vi "Teleop.vi"(10 "Match Info":T1={"Autonomous Elapsed Seconds"=0.0, "TeleOp Elapsed Seconds"=0.0, "Disabled Elapsed Seconds"=0.0, "Visited Autonomous"=FALSE, "Visited TeleOp"=FALSE, "Visited Disabled"=FALSE, "Autonomous Settings"={"Autonomous Style"=enum."Independent", "VI Refnum"=refnum}}, 11 "Call Context":T2) -> ()   [LabVIEW 2013]
doc: "This VI is called for each TeleOp packet received from the DS where the robot is not disabled. It is often used to read from the joysticks and update I/O or to update setpoints for timed control loops. It should complete and return within 20 milliseconds or it may miss DS packets."
uses:
  <vilib>/Rock Robotics/WPI/DriverStation/WPI_DriverStationDerivedRobotMode.ctl
  <vilib>/Rock Robotics/WPI/DriverStation/WPI_DriverStationMatch Info.ctl
  Robot Global Data.vi
  <vilib>/Rock Robotics/WPI/Joystick/WPI_JoystickGetSetRefNum.vi
  <vilib>/Rock Robotics/WPI/RobotDrive/WPI_RobotDriveGetSetRefNum.vi
  <vilib>/Rock Robotics/WPI/RobotDrive/WPI_RobotDriveArcadeDrive_Standard(NoSaturation).vi
panel:
  out "Angular Rate":dbl
  out "Angle":dbl
  out "Robot Moving?":bool
  out "Motor Values":dbl[](array[numeric])
  out "Numeric 1":dbl(slide) scale=0.0..100.0
  out "Boolean 2":bool
  out "Boolean 1":bool
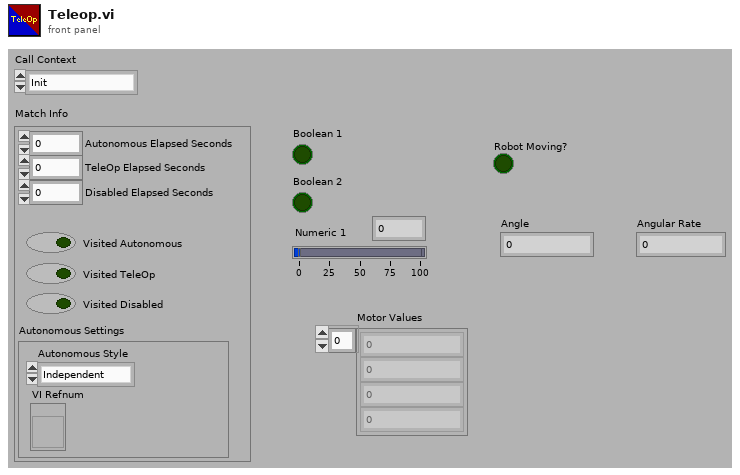
[diagram p1: front panel]
types:
  T1 = typedef "WPI_DriverStationMatch Info.ctl" = cluster{"Autonomous Elapsed Seconds":dbl, "TeleOp Elapsed Seconds":dbl, "Disabled Elapsed Seconds":dbl, "Visited Autonomous":bool, "Visited TeleOp":bool, "Visited Disabled":bool, "Autonomous Settings":cluster{"Autonomous Style":enum16{"Iterative", "Independent"}, "VI Refnum":refnum<vi>}}
  T2 = typedef "WPI_DriverStationDerivedRobotMode.ctl" = enum16{"Init", "Execute", "Stop"}
  T3 = typedef "WPI_JoystickDevRef.ctl" = cluster{"Device":T4}
  T4 = typedef "WPI_JoystickDeviceEnum.ctl" = enum16{"USB 1", "USB 2", "USB 3", "USB 4", "Kinect 1", "Kinect 2"}
  T5 = typedef "WPI_GyroDevRef.ctl" = cluster{"DevStatus":errorcluster, "Analog Module":T6, "Analog Channel":T7, "Offset":dbl, "Gain (VoltsPerDegree/Second)":dbl}
  T6 = typedef "FPGA_TypedefAnalogModule.ctl" = enum16{"Analog Module 1", "Analog Module 2"}
  T7 = typedef "FPGA_AIChannel.ctl" = enum8{"AI 1", "AI 2", "AI 3", "AI 4", "AI 5", "AI 6", "AI 7", "AI 8", "Invalid"}
  T8 = typedef "WPI_JoystickButtonState.ctl" = cluster{"Button 1":bool, "Button 2":bool, "Button 3":bool, "Button 4":bool, "Button 5":bool, "Button 6":bool, "Button 7":bool, "Button 8":bool, "Button 9":bool, "Button 10":bool, "Button 11":bool, "Button 12":bool}
  T9 = cluster{"axis 1 (x)":dbl, "axis 2 (y)":dbl, "axis 3 (throttle)":dbl, "axis 4":dbl, "axis 5":dbl, "axis 6":dbl}
  T10 = typedef "WPI_RobotDriveDevRef.ctl" = cluster{"DevStatus":errorcluster, "Motors[]":T11[], "Square Inputs":bool, "Max Output":dbl, "Isochronous":bool}
  T11 = typedef "WPI_MotorControlDeviceRef.ctl" = cluster{"DeviceStatus":errorcluster, "Type":enum16{"PWM", "CAN"}, "PWM":cluster{"Digital Module":T12, "PWM Channel":T13, "DeadBand":T14}, "CAN":cluster{"Device Number":u8, "Control Mode":T15, "Semaphore":T16, "Max Vout":dbl}, "Invert":bool, "TransformRef":T17, "InvTransformRef":T17}
  T12 = typedef "FPGA_TypedefDigitalModule.ctl" = enum16{"Digital Module 1", "Digital Module 2"}
  T13 = typedef "FPGA_DIOPWMChannel.ctl" = enum8{"PWM 1", "PWM 2", "PWM 3", "PWM 4", "PWM 5", "PWM 6", "PWM 7", "PWM 8", "PWM 9", "PWM 10", "Invalid"}
  T14 = typedef "WPI_PWMDeadband.ctl" = cluster{"Name":string, "maxPositivePwm":i32, "minPositivePwm":i32, "centerPwm":i32, "maxNegativePwm":i32, "minNegativePwm":i32, "angularRange":u16}
  T15 = typedef "WPI_CANJaguar_ControlMode.ctl" = enum8{"Percent VBus", "Current", "Speed", "Position", "Voltage"}
  T16 = typedef "Semaphore RefNum" = refnum<k1>
  T17 = typedef "WPI_PWMTransform_ConPane.ctl" = refnum<vi>
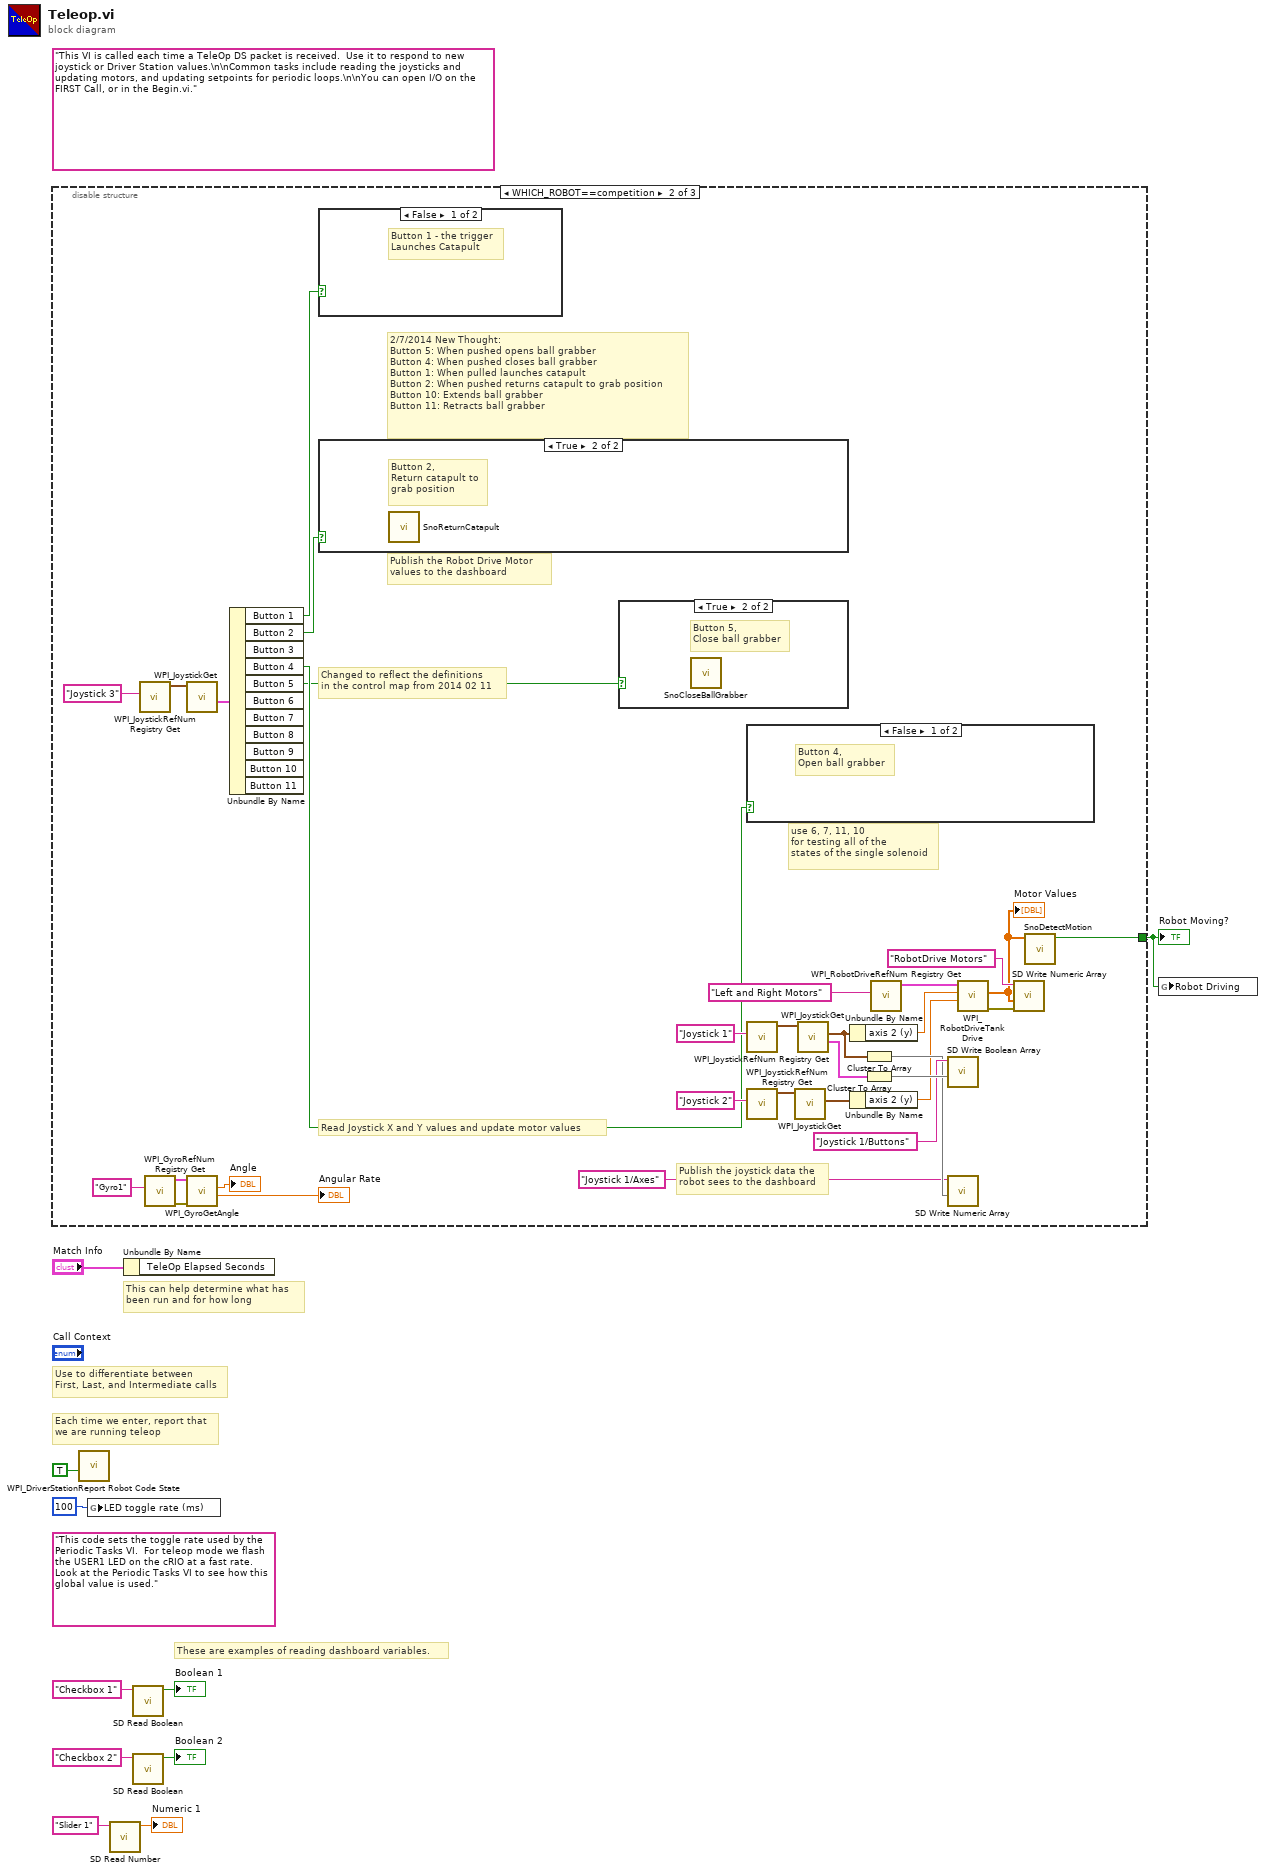
[diagram p0: block diagram]
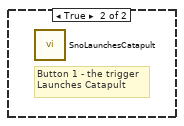
[diagram p4: hidden frame]
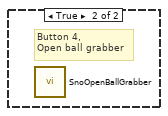
[diagram p5: hidden frame]
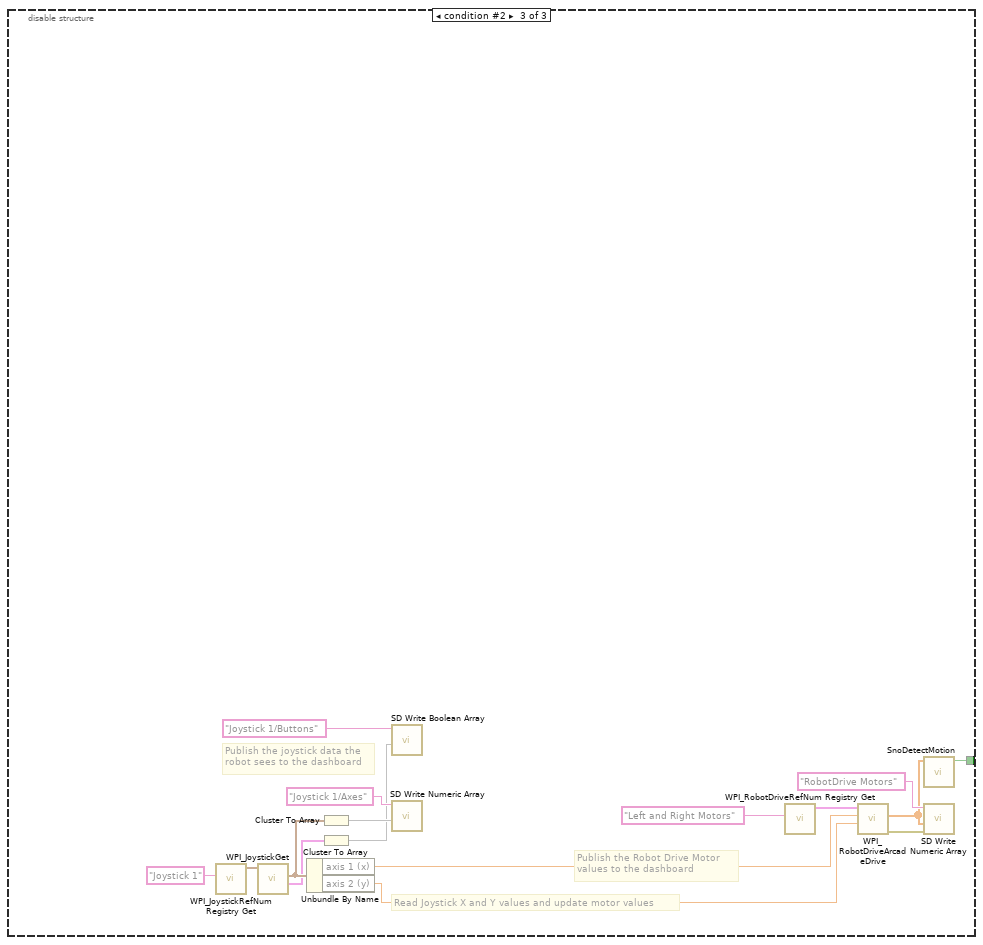
[diagram p7: hidden frame]
diagram:
  (unwired) "This code sets the toggle rate used by the Periodic Tasks VI.  For teleop mode we flash the USER1 LED on the cRIO at a fast rate.  Look at the Periodic Tasks VI to see how this global value is used."
  (unwired) "This VI is called each time a TeleOp DS packet is received.  Use it to respond to new joystick or Driver Station values.\n\nCommon tasks include reading the joysticks and updating motors, and updating setpoints for periodic loops.\n\nYou can open I/O on the FIRST Call, or in the Begin.vi."
  # "These are examples of reading dashboard variables."
  # "Each time we enter, report that\nwe are running teleop"
  # "Use to differentiate between\nFirst, Last, and Intermediate calls"
  # "This can help determine what has\nbeen run and for how long"
  n1 = disable-structure shown="WHICH_ROBOT==competition" {
    disable-tunnel: [_ w16 w42] -> w1
    frame condition #0 {
    }
    frame condition #1 (active) {
      # "use 6, 7, 11, 10\nfor testing all of the\nstates of the single solenoid"
      # "Changed to reflect the definitions\nin the control map from 2014 02 11"
      # "2/7/2014 New Thought:\nButton 5: When pushed opens ball grabber\nButton 4: When pushed closes ball grabber\nButton 1: When pulled launches catapult\nButton 2: When pushed returns catapult to grab position\nButton 10: Extends ball grabber\nButton 11: Retracts ball grabber"
      # "Publish the Robot Drive Motor\nvalues to the dashboard"
      # "Publish the joystick data the\nrobot sees to the dashboard"
      # "Read Joystick X and Y values and update motor values"
      n2 = call <vilib>:"WPI_JoystickRefNum Registry Get.vi"("refnum name"="Joystick 3") -> ("JoystickDevRef"=w25:T3)  [unwired: 1 in, 9 out]
      n3 = call <vilib>:"WPI_GyroRefNum Registry Get.vi"("refnum name"="Gyro1") -> ("error out"=w13:errorcluster, "GyroDevRef"=w14:T5)  [unwired: 9 in]
      n4 = call <vilib>:"WPI_JoystickGet.vi"("JoystickDevRef"=w25) -> ("Buttons"=w23:T8)  [unwired: 1 in, 5 out]
      n5 = call <vilib>:"WPI_GyroGetAngle.vi"("error in (no error)"=w13, "GyroDevRef"=w14) -> ("Angular Rate"=→"Angular Rate":dbl, "Angle"=→"Angle":dbl)  [unwired: 6 in, 2 out]
      n6 = Unbundle By Name(w23) -> ("Button 1"=w19:bool, "Button 2"=w18:bool, "Button 4"=w22:bool, "Button 5"=w21:bool)  [unwired: 7 out]
      n7 = case shown="False" w19 {
        frame False {
          # "Button 1 - the trigger\nLaunches Catapult"
        }
        frame True {
          # "Button 1 - the trigger\nLaunches Catapult"
          n8 = call "SnoLaunchesCatapult.vi"() -> ()  [unwired: 12 in]
        }
      }
      n9 = case shown="True" w18 {
        frame False {
          # "Button 2,\nReturn catapult to\ngrab position"
        }
        frame True {
          # "Button 2,\nReturn catapult to\ngrab position"
          n10 = call "SnoReturnCatapult.vi"() -> ()  [unwired: 12 in]
        }
      }
      n11 = case shown="True" w21 {
        frame False {
          # "Button 5,\nClose ball grabber"
        }
        frame True {
          # "Button 5,\nClose ball grabber"
          n12 = call "SnoCloseBallGrabber.vi"() -> ()  [unwired: 1 in, 2 out]
        }
      }
      n13 = case shown="False" w22 {
        frame False {
          # "Button 4,\nOpen ball grabber"
        }
        frame True {
          # "Button 4,\nOpen ball grabber"
          n14 = call "SnoOpenBallGrabber.vi"() -> ()  [unwired: 1 in, 1 out]
        }
      }
      n15 = call <vilib>:"WPI_JoystickRefNum Registry Get.vi"("refnum name"="Joystick 1") -> ("JoystickDevRef"=w39:T3)  [unwired: 1 in, 9 out]
      n16 = call <vilib>:"WPI_JoystickRefNum Registry Get.vi"("refnum name"="Joystick 2") -> ("JoystickDevRef"=w31:T3)  [unwired: 1 in, 9 out]
      n17 = call <vilib>:"WPI_JoystickGet.vi"("JoystickDevRef"=w31) -> ("Axes"=w30:T9)  [unwired: 1 in, 5 out]
      n18 = call <vilib>:"WPI_JoystickGet.vi"("JoystickDevRef"=w39) -> ("Buttons"=w20:T8, "Axes"=w36:T9)  [unwired: 1 in, 4 out]
      n19 = Unbundle By Name(w36) -> ("axis 2 (y)"=w28:dbl)
      n20 = Unbundle By Name(w30) -> ("axis 2 (y)"=w27:dbl)
      n21 = Cluster To Array(cluster=w36) -> (array=w35:dbl[])
      n22 = Cluster To Array(cluster=w20) -> (array=w38:bool[])
      n23 = call <vilib>:"WPI_RobotDriveRefNum Registry Get.vi"("refnum name"="Left and Right Motors") -> ("RobotDriveDevRef"=w29:T10)  [unwired: 1 in, 9 out]
      n24 = call <vilib>:"SD Write Boolean Array.vi"("Boolean Array"=w38, "Name"="Joystick 1/Buttons") -> ()  [unwired: 8 in, 2 out]
      n25 = call <vilib>:"SD Write Numeric Array.vi"("Numeric Array"=w35, "Name"="Joystick 1/Axes") -> ()  [unwired: 8 in, 2 out]
      n26 = call <vilib>:"WPI_RobotDriveTankDrive.vi"("Right axis value"=w27, "Left axis value"=w28, "RobotDriveDevRef"=w29) -> ("error out"=w26:errorcluster, "Motor Values"=w17:dbl[])  [unwired: 6 in, 1 out]
      "Motor Values" <- w17
      n27 = call <vilib>:"SD Write Numeric Array.vi"("error in"=w26, "Numeric Array"=w17, "Name"="RobotDrive Motors") -> ()  [unwired: 7 in, 2 out]
      n28 = call "SnoDetectMotion.vi"("Motor Values"=w17) -> ("Boolean"=w16:bool)  [unwired: 10 in]
    }
    frame condition #2 {
      # "Publish the Robot Drive Motor\nvalues to the dashboard"
      # "Publish the joystick data the\nrobot sees to the dashboard"
      # "Read Joystick X and Y values and update motor values"
      n29 = call <vilib>:"WPI_JoystickRefNum Registry Get.vi"("refnum name"="Joystick 1") -> ("JoystickDevRef"=w46:T3)  [unwired: 1 in, 9 out]
      n30 = call <vilib>:"WPI_JoystickGet.vi"("JoystickDevRef"=w46) -> ("Buttons"=w47:T8, "Axes"=w50:T9)  [unwired: 1 in, 4 out]
      n31 = Unbundle By Name(w50) -> ("axis 1 (x)"=w56:dbl, "axis 2 (y)"=w57:dbl)
      n32 = Cluster To Array(cluster=w50) -> (array=w51:dbl[])
      n33 = Cluster To Array(cluster=w47) -> (array=w48:bool[])
      n34 = call <vilib>:"SD Write Boolean Array.vi"("Boolean Array"=w48, "Name"="Joystick 1/Buttons") -> ()  [unwired: 8 in, 2 out]
      n35 = call <vilib>:"SD Write Numeric Array.vi"("Numeric Array"=w51, "Name"="Joystick 1/Axes") -> ()  [unwired: 8 in, 2 out]
      n36 = call <vilib>:"WPI_RobotDriveRefNum Registry Get.vi"("refnum name"="Left and Right Motors") -> ("RobotDriveDevRef"=w54:T10)  [unwired: 1 in, 9 out]
      n37 = call-poly <vilib>:"WPI_RobotDriveArcadeDrive.vi"("Y axis value"=w57, "X axis value"=w56, "RobotDriveDevRef"=w54) -> ("error out"=w55:errorcluster, "Motor Values"=w43:dbl[])  [unwired: 6 in, 1 out]
      n38 = call "SnoDetectMotion.vi"("Motor Values"=w43) -> ("Boolean"=w42:bool)  [unwired: 10 in]
      n39 = call <vilib>:"SD Write Numeric Array.vi"("error in"=w55, "Numeric Array"=w43, "Name"="RobotDrive Motors") -> ()  [unwired: 7 in, 2 out]
    }
  }
  "Robot Moving?" <- w1
  n40 = call <vilib>:"WPI_DriverStationReport Robot Code State.vi"("TeleOp"=TRUE ("Autonomous")) -> ()  [unwired: 10 in, 1 out]
  n41 = global write "Robot Global Data.vi" "LED toggle rate (ms)"(u32 100 ("LED ms toggle rate")) -> ()
  n42 = call <vilib>:"SD Read Number.vi"("Name"="Slider 1" ("refnum name")) -> ("Numeric"=→"Numeric 1":dbl)  [unwired: 8 in, 2 out]
  n43 = Unbundle By Name("Match Info") -> ()  [unwired: 1 out]
  n44 = call <vilib>:"SD Read Boolean.vi"("Name"="Checkbox 1" ("refnum name")) -> ("Boolean"=→"Boolean 1":bool)  [unwired: 8 in, 2 out]
  n45 = call <vilib>:"SD Read Boolean.vi"("Name"="Checkbox 2" ("refnum name")) -> ("Boolean"=→"Boolean 2":bool)  [unwired: 8 in, 2 out]
  n46 = global write "Robot Global Data.vi" "Robot Driving"(w1) -> ()
